vi "Seleccion Producto.vi"(8 "error in (no error)":errorcluster, 11 "Soda Actor in":refnum<class "Soda Actor.lvclass">) -> (0 "error out":errorcluster, 3 "Soda Actor out":refnum<class "Soda Actor.lvclass">)   [LabVIEW 2020, in "Soda Actor.lvlib" / "Soda Actor.lvclass"]
uses:
  Soda Actor.lvclass
  C:/Program Files (x86)/National Instruments/LabVIEW 2020/vi.lib/ActorFramework/Actor/Actor.lvclass
  <vilib>/ActorFramework/Actor/Actor.lvclass/Actor.ctl
  Soda Actor.lvclass/Soda Actor.ctl
  MSG Messages/Update MSG Msg/Update MSG Msg.lvclass/Update MSG Msg.ctl
  <vilib>/ActorFramework/Message Enqueuer/Message Enqueuer.lvclass/Message Enqueuer.ctl
  <vilib>/ActorFramework/Message Enqueuer/Enqueue.vi
  MSG Messages/Update MSG Msg/Update MSG Msg.lvclass
  C:/Program Files (x86)/National Instruments/LabVIEW 2020/vi.lib/ActorFramework/Message/Message.lvclass
  <vilib>/ActorFramework/Message Priority Queue/Priority Enqueue.vi
  <vilib>/ActorFramework/Actor/Actor.lvclass
panel:
  out "Set Products":string[][](array[string])
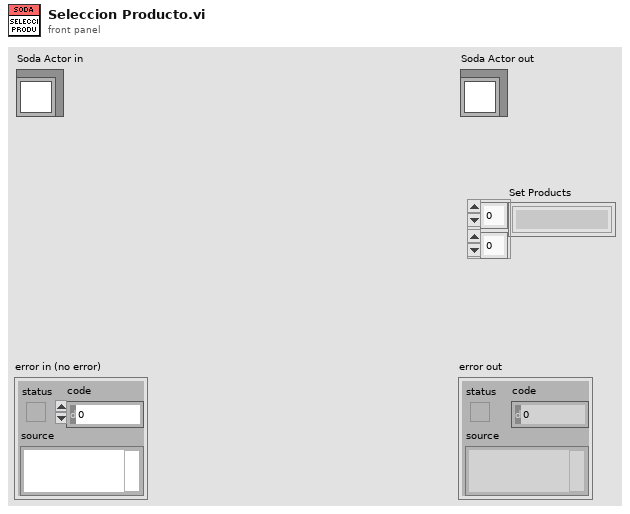
[diagram p1: front panel]
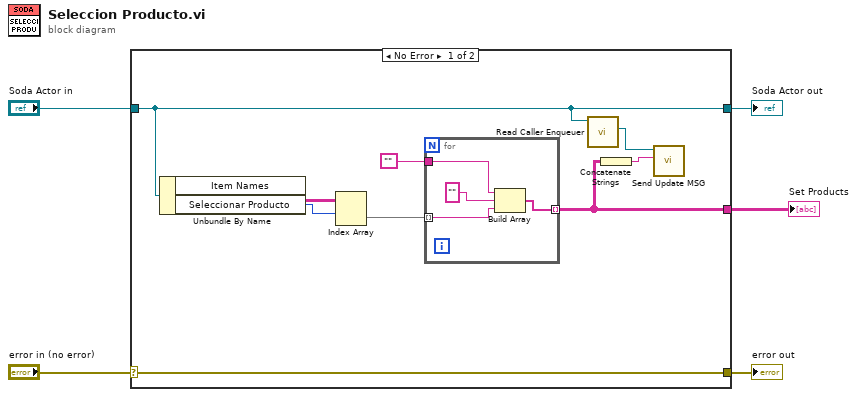
[diagram p0: block diagram]
diagram:
  n1 = case shown="No Error" "error in (no error)" {
    selector: "error in (no error)" -> [w14 w20]
    tunnel: [w14 w20] -> w4
    tunnel: [w8 w19] -> w2
    tunnel: "Soda Actor in" -> [w8 w19]
    tunnel: [w10 _] -> w1
    frame No Error {
      n2 = Unbundle By Name(w8) -> ("Item Names"=w13:string[][], "Seleccionar Producto"=w6:enum16{"Coca", "Fanta", "Manzanita", "Ciel"})
      n3 = Index Array(array=w13, index (row)=w6) -> (element=w11:string[])  [unwired: 1 in]
      n4 = for {
        tunnel: "" -> [w18]
        tunnel: w11 -> [w16] mode=indexing
        tunnel: [w15] -> w10 mode=indexing
        n5 = Build Array(w18, "" ("element"), w16) -> (w15:string[])
      }
      n6 = call <vilib>:"Read Caller Enqueuer.vi"("Actor"=w8) -> ("Caller Enqueuer"=w7:refnum<class "Message Enqueuer.lvclass">)  [unwired: 10 in]
      n7 = Concatenate Strings(w10) -> (w9:string)
      n8 = call "Send Update MSG.vi"("Update message"=w9, "Message Enqueuer"=w7) -> ()  [unwired: 8 in, 2 out]
    }
    frame Error {
    }
  }
  "error out" <- w4
  "Soda Actor out" <- w2
  "Set Products" <- w1
